vi "Urgency Sort.vi"(11 "list in":T1[](array[typedef]) {"Creation Date" format="%<%x>T"; "Last Updated" format="%<%x>T"}) -> (3 "Array":T1[](array[typedef]) {"Creation Date" format="%<%x>T"; "Last Updated" format="%<%x>T"})   [LabVIEW 2018]
uses:
  Type Defs/SR Cluster.ctl
  Type Defs/SR Status.ctl
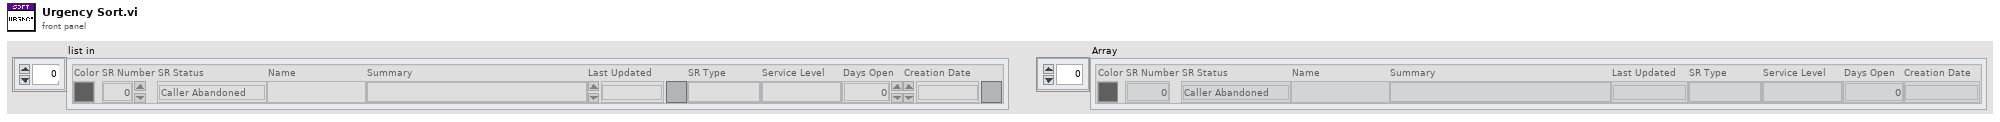
[diagram p1: front panel]
types:
  T1 = typedef "SR Cluster.ctl" = cluster{"Color":u32, "SR Number":i32, "SR Status":T2, "Name":string, "Summary":string, "Last Updated":timestamp, "SR Type":string, "Service Level":string, "Days Open":dbl, "Creation Date":timestamp}
  T2 = typedef "SR Status.ctl" = enum16{"Caller Abandoned", "Created in Error", "Expired", "Forum Resolved AE", "Forum Resolved Customer", "IN WORK", "IN WORK Collab with AES", "IN WORK Collab with PSE", "IN WORK Collab with SE", "IN WORK Customer Added Note", "IN WORK Escalation", "IN WORK Wait on Customer", "Open", "Potentially Resolved", "Presumed Resolved", "RMA Approved for Return", "RMA Closed", "RMA Closed - DOA", "RMA In Progress", "RMA Open", "RMA Waiting on Customer", "Resolved", "Passed Off"}
  T3 = cluster{i32, string, dbl, dbl, "SR Cluster":T1}[]
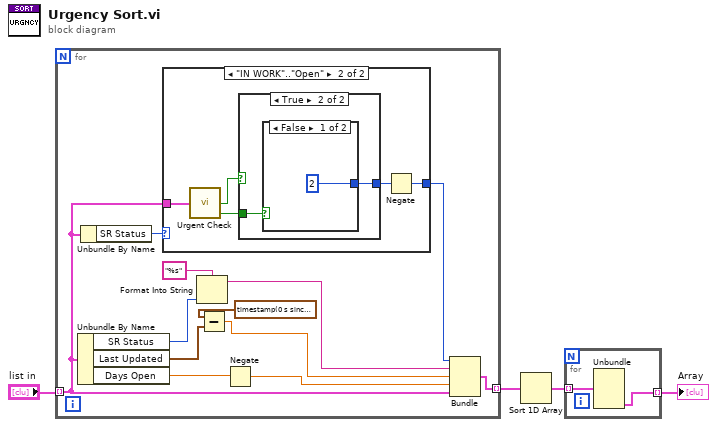
[diagram p0: block diagram]
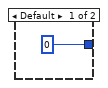
[diagram p2: hidden frame]
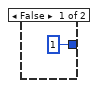
[diagram p3: hidden frame]
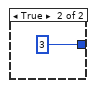
[diagram p4: hidden frame]
diagram:
  n1 = for {
    tunnel: "list in" -> [w8] mode=indexing
    tunnel: [w16] -> w1 mode=indexing
    n2 = Unbundle By Name(w8) -> ("SR Status"=w15:T2, "Last Updated"=w10:timestamp, "Days Open"=w6:dbl)
    n3 = Unbundle By Name(w8) -> ("SR Status"=w7:T2)
    n4 = case shown="\"IN WORK\"..\"Open\"" w7 {
      tunnel: w8 -> [_ w22]
      tunnel: [0 w18] -> w9
      frame Default {
      }
      frame "IN WORK".."Open" {
        n5 = call "Urgent Check.vi"("SR Cluster"=w22) -> ("Passed Due?"=w20:bool, "Answer Today?"=w21:bool)  [unwired: 3 in]
        n6 = case shown="True" w21 {
          tunnel: w20 -> [_ w25]
          tunnel: [1 w24] -> w19
          frame False {
          }
          frame True {
            n7 = case shown="False" w25 {
              tunnel: [2 3] -> w24
              frame False {
              }
              frame True {
              }
            }
          }
        }
        n8 = Negate(x=w19) -> (-x=w18:i32)
      }
    }
    n9 = Format Into String(format string="%s", w15) -> (resulting string=w12:string)  [unwired: 2 in, 1 out]
    n10 = Subtract(x=timestamp(0 s since 1904-01-01), y=w10) -> (x-y=w11:dbl)
    n11 = Negate(x=w6) -> (-x=w5:dbl)
    n12 = Bundle(w9, w12, w11, w5, "SR Cluster"=w8) -> (w16:cluster{i32, string, dbl, dbl, "SR Cluster":T1})  [unwired: 1 in]
  }
  n13 = Sort 1D Array(array=w1) -> (sorted array=w2:T3)
  n14 = for {
    tunnel: w2 -> [w29] mode=indexing
    tunnel: [w28] -> w4 mode=indexing
    n15 = Unbundle(w29) -> ("SR Cluster"=w28:T1)  [unwired: 4 out]
  }
  "Array" <- w4
